vi "Library Path.vi"() -> (2 "Library Path":path)   [LabVIEW 2020]
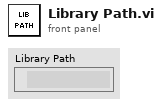
[diagram p1: front panel]
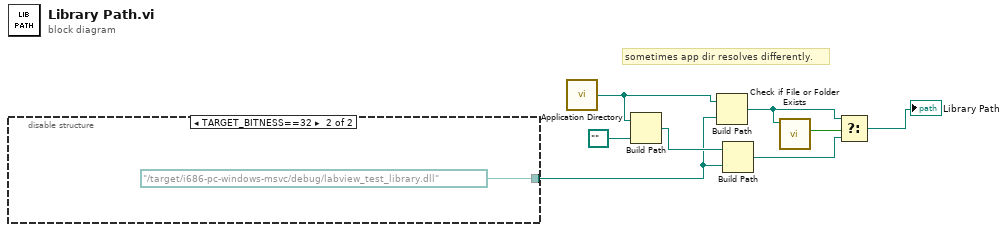
[diagram p0: block diagram]
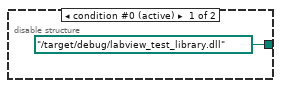
[diagram p2: hidden frame]
diagram:
  # "sometimes app dir resolves differently."
  n1 = disable-structure shown="TARGET_BITNESS==32" {
    disable-tunnel: [path "../target/debug/labview_test_library.dll" path "../target/i686-pc-windows-msvc/debug/labview_test_library.dll"] -> w5
    frame condition #0 (active) {
    }
    frame condition #1 {
    }
  }
  n2 = call <vilib>:"Application Directory.vi"() -> ("Application Directory"=w8:path)
  n3 = Build Path(base path=w8, name or relative path=path "..") -> (appended path=w6:path)
  n4 = Build Path(base path=w8, name or relative path=w5) -> (appended path=w2:path)
  n5 = Build Path(base path=w6, name or relative path=w5) -> (appended path=w4:path)
  n6 = call <vilib>:"Check if File or Folder Exists.vi"("path"=w2) -> ("file or folder exists?"=w1:bool)  [unwired: 8 in, 2 out]
  n7 = Select(t=w2, s=w1, f=w4) -> (s? t:f=→"Library Path":path)
